vi "Control Message Loop.vi"(8 "error in (no error)":errorcluster, 11 "Message Queues":T1) -> (0 "error out":errorcluster)   [LabVIEW 2015, in "Control.lvlib"]
uses:
  Control.lvlib
  Settings/Settings.ctl
  Settings/Settings.lvlib
  Support/Message Queue/Message Queue.lvlib
  <vilib>/ErrorRing/Error Ring.xnode
  <vilib>/Utility/error.llb/Error Cluster From Error Code.vi
  Settings/Scope settings.ctl
  Settings/PFC Control settings.ctl
  Acquisition/PI Compensator.ctl
  Support/Message Queue/Message Cluster.ctl
  Support/Message Queue/All Message Queues.ctl
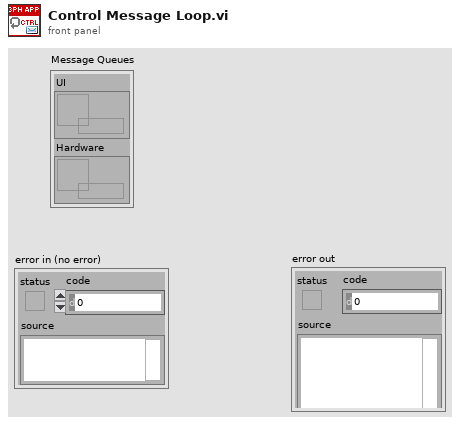
[diagram p1: front panel]
types:
  T1 = typedef "Message Queue.lvlib/All Message Queues.ctl" = cluster{"UI":refnum<queue>, "Hardware":refnum<queue>}
  T2 = typedef "Settings.lvlib/Settings.ctl" = cluster{"HW Refnum":refnum<visa-resource-name>, "Control settings":T3, "Scope settings":T5}
  T3 = typedef "Settings.lvlib/PFC Control settings.ctl" = cluster{"FSM status":enum8{"Stopped", "Running"}, "Voltage control ena":bool, "Vea":sgl, "Voltage Ctrl bypass":bool, "PI Voltage control":T4, "Current Ctrl bypass":bool, "PI Current control":T4, "PFC 3rd Harmonic":bool, "PFC Output enable":bool}
  T4 = typedef "Settings.lvlib/PI Compensator.ctl" = cluster{"Ref_val":sgl, "Kp":sgl, "Ki2":sgl, "Out_min":sgl, "Out_max":sgl}
  T5 = typedef "Settings.lvlib/Scope settings.ctl" = cluster{"run_stop":bool, "single mode":bool, "Trigger mode":enum16{"Auto", "Rising Edge", "Falling Edge", "Both Edges"}, "Trigger source":u16, "trigger level":dbl, "acq width":dbl}
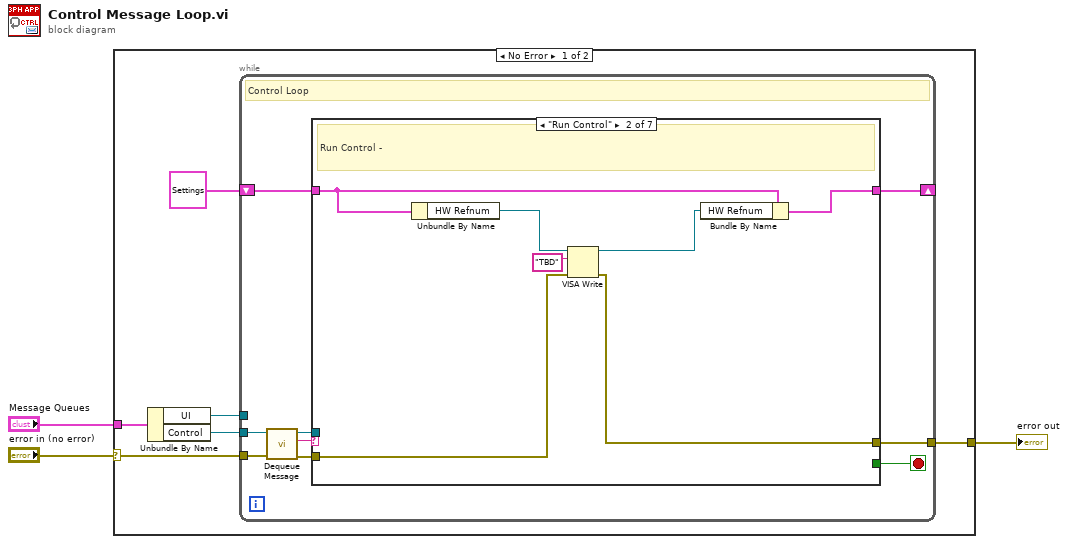
[diagram p0: block diagram]
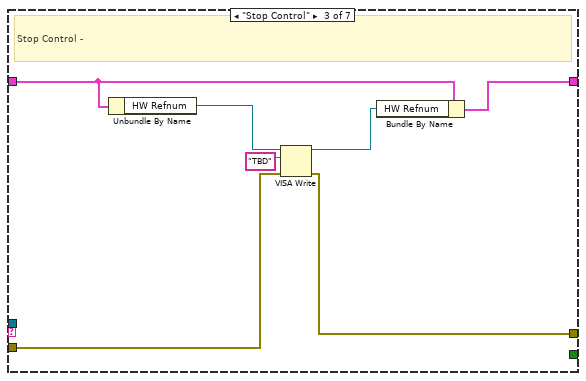
[diagram p3: hidden frame]
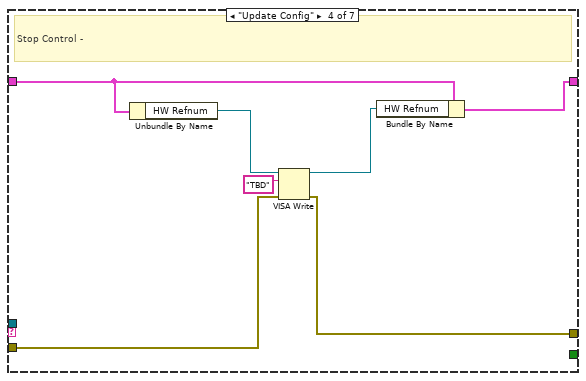
[diagram p4: hidden frame]
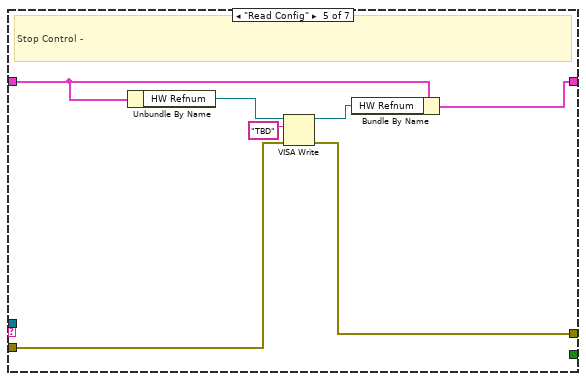
[diagram p5: hidden frame]
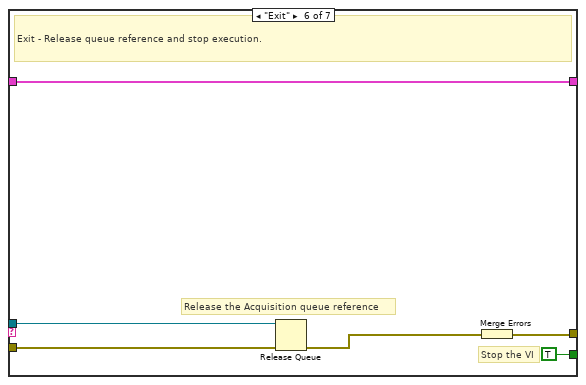
[diagram p6: hidden frame]
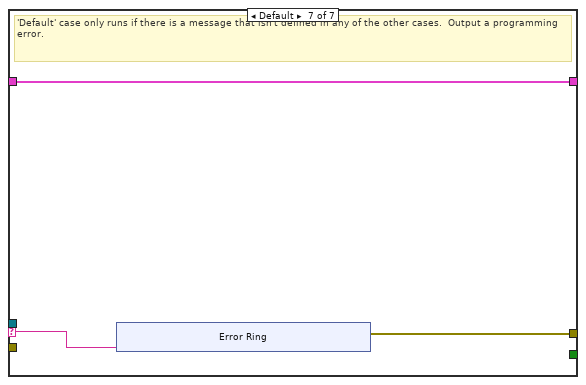
[diagram p7: hidden frame]
diagram:
  n1 = case shown="No Error" "error in (no error)" {
    selector: "error in (no error)" -> [w6 w65]
    tunnel: "Message Queues" -> [w9 _]
    tunnel: [w5 w65] -> w1
    frame No Error {
      n2 = Unbundle By Name(w9) -> ("UI"=w8:refnum<queue>, "Control"=w7:refnum<queue>)
      n3 = while {
        tunnel: w8 -> [_]
        tunnel: w7 -> [w18]
        tunnel: w6 -> [w16]
        tunnel: [w14] -> w5
        shift-right: [w10] -> _
        shift-left: T2 {"HW Refnum"="", "Control settings"={"FSM status"=enum."Running", "Voltage control ena"=FALSE, "Vea"=0.0, "Voltage Ctrl bypass"=FALSE, "PI Voltage control"={"Ref_val"=0.0, "Kp"=0.0, "Ki2"=0.0, "Out_min"=0.0, "Out_max"=0.0}, "Current Ctrl bypass"=FALSE, "PI Current control"={"Ref_val"=0.0, "Kp"=0.0, "Ki2"=0.0, "Out_min"=0.0, "Out_max"=0.0}, "PFC 3rd Harmonic"=FALSE, "PFC Output enable"=FALSE}, "Scope settings"={"run_stop"=FALSE, "single mode"=FALSE, "Trigger mode"=enum."Auto", "Trigger source"=0, "trigger level"=0.0, "acq width"=0.0}} ("Data Cluster") -> [w11]
        stop <- w15 stop-if-true
        # "Control Loop"
        n4 = call "Dequeue Message.vi"("error in (no error)"=w16, "Message Queue"=w18) -> ("error out"=w13:errorcluster, "Message"=w17:string, "dup Message Queue"=w12:refnum<queue>)  [unwired: 6 in, 1 out]
        n5 = case shown="\"Run Control\"" w17 {
          selector: w17 -> [_ _ _ _ _ _ w57]
          tunnel: [w19 w24 w31 w38 w45 w52 w56] -> w14
          tunnel: [_ _ _ _ _ TRUE _] -> w15
          tunnel: w13 -> [w19 w25 w32 w39 w46 w51 _]
          tunnel: w12 -> [_ _ _ _ _ w50 _]
          tunnel: w11 -> [w20 w22 w30 w35 w42 w49 w55]
          tunnel: [w20 w21 w28 w36 w43 w49 w55] -> w10
          frame "Initialize" {
          }
          frame "Run Control" {
            # "Run Control -"
            n6 = Unbundle By Name(w22) -> ("HW Refnum"=w26:refnum<visa-resource-name>)
            n7 = VISA Write(VISA resource name=w26, write buffer="TBD", error in (no error)=w25) -> (VISA resource name out=w23:refnum<visa-resource-name>, error out=w24:errorcluster)  [unwired: 1 out]
            n8 = Bundle By Name(cluster=w22, "HW Refnum"=w23) -> (w21:T2)
          }
          frame "Stop Control" {
            # "Stop Control -"
            n9 = Unbundle By Name(w30) -> ("HW Refnum"=w33:refnum<visa-resource-name>)
            n10 = VISA Write(VISA resource name=w33, write buffer="TBD", error in (no error)=w32) -> (VISA resource name out=w29:refnum<visa-resource-name>, error out=w31:errorcluster)  [unwired: 1 out]
            n11 = Bundle By Name(cluster=w30, "HW Refnum"=w29) -> (w28:T2)
          }
          frame "Update Config" {
            # "Stop Control -"
            n12 = Unbundle By Name(w35) -> ("HW Refnum"=w40:refnum<visa-resource-name>)
            n13 = VISA Write(VISA resource name=w40, write buffer="TBD", error in (no error)=w39) -> (VISA resource name out=w37:refnum<visa-resource-name>, error out=w38:errorcluster)  [unwired: 1 out]
            n14 = Bundle By Name(cluster=w35, "HW Refnum"=w37) -> (w36:T2)
          }
          frame "Read Config" {
            # "Stop Control -"
            n15 = Unbundle By Name(w42) -> ("HW Refnum"=w47:refnum<visa-resource-name>)
            n16 = VISA Write(VISA resource name=w47, write buffer="TBD", error in (no error)=w46) -> (VISA resource name out=w44:refnum<visa-resource-name>, error out=w45:errorcluster)  [unwired: 1 out]
            n17 = Bundle By Name(cluster=w42, "HW Refnum"=w44) -> (w43:T2)
          }
          frame "Exit" {
            # "Release the Acquisition queue reference"
            # "Stop the VI"
            # "Exit - Release queue reference and stop execution."
            n18 = Release Queue(queue=w50, error in (no error)=w51) -> (error out=w54:errorcluster)  [unwired: 1 in, 2 out]
            n19 = Merge Errors(w54) -> (w52:errorcluster)
          }
          frame Default {
            # "'Default' case only runs if there is a message that isn't defined in any of the other cases.  Output a programming error."
            n20 = xnode "Error Ring"("parameter 0"=w57) -> ("error out"=w56:errorcluster)
          }
        }
      }
    }
    frame Error {
    }
  }
  "error out" <- w1
